vi "draw.notes.vi"(8 "error in (no error)":errorcluster, 11 "midi-ui in":refnum<class "midi-ui.lvclass">) -> (0 "error out":errorcluster, 3 "midi-ui out":refnum<class "midi-ui.lvclass">)   [LabVIEW 2020, in "midi-ui.lvclass"]
uses:
  midi-ui.lvclass
  midi-ui.lvclass/midi-ui.ctl
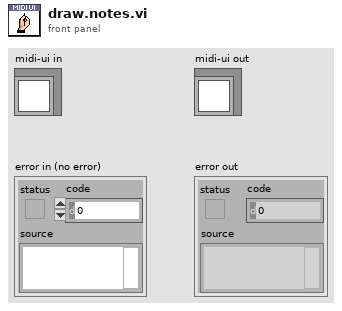
[diagram p1: front panel]
types:
  T1 = map{string, cluster{"Note On":picture, "Note Off":picture}}
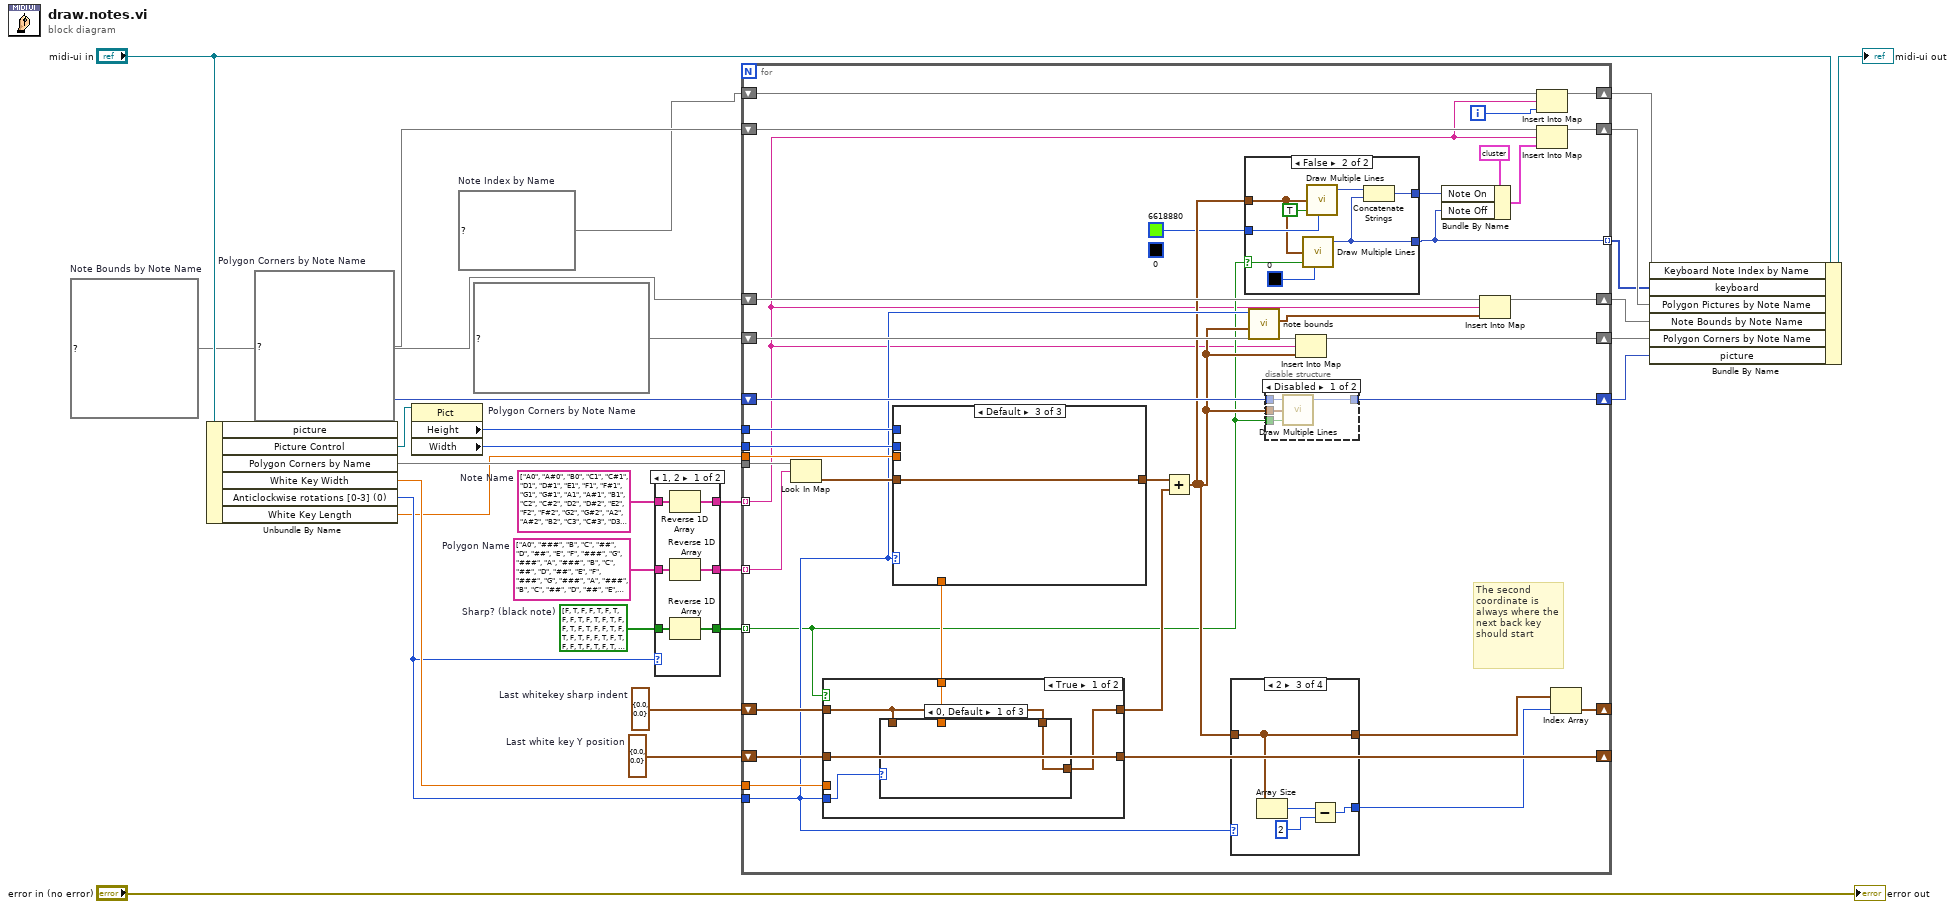
[diagram p0: block diagram]
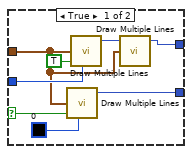
[diagram p4: hidden frame]
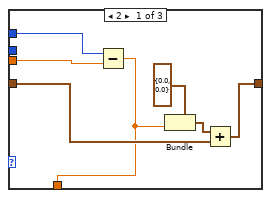
[diagram p5: hidden frame]
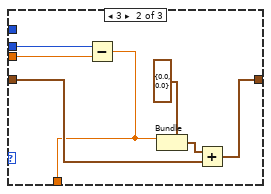
[diagram p6: hidden frame]
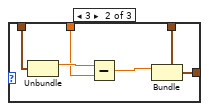
[diagram p7: hidden frame]
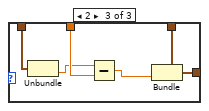
[diagram p8: hidden frame]
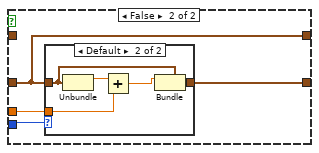
[diagram p9: hidden frame]
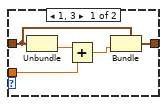
[diagram p10: hidden frame]
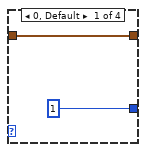
[diagram p11: hidden frame]
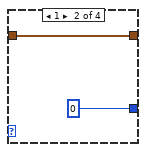
[diagram p12: hidden frame]
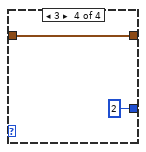
[diagram p13: hidden frame]
diagram:
  w2 = map{string, i32} {}  # Note Index by Name
  w5 = T1 {}  # Polygon Corners by Note Name
  w7 = map{string, cluster{"max":dbl, "min":dbl}} {}  # Note Bounds by Note Name
  w22 = bool[] [FALSE, TRUE, FALSE, FALSE, TRUE, FALSE, TRUE, FALSE, FALSE, TRUE, FALSE, TRUE, FALSE, TRUE, FALSE, FALSE, TRUE, FALSE, TRUE, FALSE, FALSE, TRUE, FALSE, TRUE, FALSE, TRUE, FALSE, FALSE, TRUE, FALSE, TRUE, FALSE, FALSE, TRUE, FALSE, TRUE, FALSE, TRUE, FALSE, FALSE, TRUE, FALSE, TRUE, FALSE, FALSE, TRUE, FALSE, TRUE, FALSE, TRUE, FALSE, FALSE, TRUE, FALSE, TRUE, FALSE, FALSE, TRUE, FALSE, TRUE, FALSE, TRUE, FALSE, FALSE, TRUE, FALSE, TRUE, FALSE, FALSE, TRUE, FALSE, TRUE, FALSE, TRUE, FALSE, FALSE, TRUE, FALSE, TRUE, FALSE, FALSE, TRUE, FALSE, TRUE, FALSE, TRUE, FALSE, FALSE]  # Sharp? (black note)
  w23 = string[] ["A0", "###", "B", "C", "##", "D", "##", "E", "F", "###", "G", "###", "A", "###", "B", "C", "##", "D", "##", "E", "F", "###", "G", "###", "A", "###", "B", "C", "##", "D", "##", "E", "F", "###", "G", "###", "A", "###", "B", "C", "##", "D", "##", "E", "F", "###", "G", "###", "A", "###", "B", "C", "##", "D", "##", "E", "F", "###", "G", "###", "A", "###", "B", "C", "##", "D", "##", "E", "F", "###", "G", "###", "A", "###", "B", "C", "##", "D", "##", "E", "F", "###", "G", "###", "A", "###", "B", "C8"]  # Polygon Name
  w24 = string[] ["A0", "A#0", "B0", "C1", "C#1", "D1", "D#1", "E1", "F1", "F#1", "G1", "G#1", "A1", "A#1", "B1", "C2", "C#2", "D2", "D#2", "E2", "F2", "F#2", "G2", "G#2", "A2", "A#2", "B2", "C3", "C#3", "D3", "D#3", "E3", "F3", "F#3", "G3", "G#3", "A3", "A#3", "B3", "C4", "C#4", "D4", "D#4", "E4", "F4", "F#4", "G4", "G#4", "A4", "A#4", "B4", "C5", "C#5", "D5", "D#5", "E5", "F5", "F#5", "G5", "G#5", "A5", "A#5", "B5", "C6", "C#6", "D6", "D#6", "E6", "F6", "F#6", "G6", "G#6", "A6", "A#6", "B6", "C7", "C#7", "D7", "D#7", "E7", "F7", "F#7", "G7", "G#7", "A7", "A#7", "B7", "C8"]  # Note Name
  w27 = map{string, cluster{"x":dbl, "y":dbl}[]} {}  # Polygon Corners by Note Name
  w28 = cluster{"x":dbl, "y":dbl} {"x"=0.0, "y"=0.0}  # Last whitekey sharp indent
  w29 = cluster{"x":dbl, "y":dbl} {"x"=0.0, "y"=0.0}  # Last white key Y position
  n1 = Unbundle By Name("midi-ui in") -> ("picture"=w9:picture, "Picture Control"=w13:refnum<vi>, "Polygon Corners by Name"=w26:map{string, cluster{"x":dbl, "y":dbl}[]}, "White Key Width"=w20:dbl, "Anticlockwise rotations [0-3] (0)"=w16:i32, "White Key Length"=w11:dbl)
  n2 = property class="Pict"(reference=w13) -> ("Height"=w12:u32, "Width"=w10:u32)  [unwired: 1 in, 2 out]
  n3 = case shown="1, 2" w16 {
    tunnel: w24 -> [w35 w38]
    tunnel: w23 -> [w34 w37]
    tunnel: w22 -> [w33 w36]
    tunnel: [w32 w38] -> w19
    tunnel: [w31 w37] -> w18
    tunnel: [w30 w36] -> w17
    frame 1, 2 {
      n4 = Reverse 1D Array(array=w35) -> (reversed array=w32:string[])
      n5 = Reverse 1D Array(array=w34) -> (reversed array=w31:string[])
      n6 = Reverse 1D Array(array=w33) -> (reversed array=w30:bool[])
    }
    frame Default {
    }
  }
  n7 = for {
    tunnel: w26 -> [w74]
    shift-right: [w64] -> w8
    shift-left: w9 -> [w75]
    tunnel: w19 -> [w42] mode=indexing
    shift-right: [w73] -> _
    shift-left: w29 -> [w72]
    shift-right: [w69] -> _
    shift-left: w28 -> [w70]
    shift-right: [w67] -> w15
    shift-left: w27 -> [w68]
    tunnel: w18 -> [w66] mode=indexing
    tunnel: w17 -> [w45] mode=indexing
    tunnel: w20 -> [w65]
    tunnel: w16 -> [w52]
    tunnel: w12 -> [w61]
    tunnel: w11 -> [w60]
    tunnel: w10 -> [w59]
    shift-right: [w54] -> w6
    shift-left: w7 -> [w55]
    shift-right: [w51] -> w4
    shift-left: w5 -> [w50]
    tunnel: [w39] -> w3 mode=indexing
    shift-right: [w43] -> w1
    shift-left: w2 -> [w44]
    i -> [w41]
    (unwired) u32 0 ("color(black)")
    # "The second coordinate is always where the next back key should start"
    n8 = Look In Map(map=w74, key=w66) -> (value=w57:cluster{"x":dbl, "y":dbl}[])  [unwired: 1 in, 1 out]
    n9 = case shown="Default" w52 {
      tunnel: [w98 w106 w111] -> w62
      tunnel: w57 -> [w100 w108 w111]
      tunnel: w61 -> [w103 _ _]
      tunnel: w60 -> [w102 w110 _]
      tunnel: w59 -> [_ w105 _]
      tunnel: [w97 w104 _] -> w56
      frame 2 {
        n10 = Subtract(x=w103, y=w102) -> (x-y=w97:dbl)
        n11 = Bundle(cluster=cluster{"x":dbl, "y":dbl} {"x"=0.0, "y"=0.0} ("coordinate"), "y"=w97) -> (w101:cluster{"x":dbl, "y":dbl})  [unwired: 1 in]
        n12 = Add(x=w101, y=w100) -> (x+y=w98:cluster{"x":dbl, "y":dbl}[])
      }
      frame 3 {
        n13 = Subtract(x=w105, y=w110) -> (x-y=w104:dbl)
        n14 = Bundle(cluster=cluster{"x":dbl, "y":dbl} {"x"=0.0, "y"=0.0} ("coordinate"), "x"=w104) -> (w109:cluster{"x":dbl, "y":dbl})  [unwired: 1 in]
        n15 = Add(x=w109, y=w108) -> (x+y=w106:cluster{"x":dbl, "y":dbl}[])
      }
      frame Default {
      }
    }
    n16 = case shown="True" w45 {
      tunnel: w72 -> [w116 w132]
      tunnel: [w116 w133] -> w73
      tunnel: [w114 w132] -> w71
      tunnel: w70 -> [w113 _]
      tunnel: w65 -> [_ w131]
      tunnel: w52 -> [w115 w130]
      tunnel: w56 -> [w112 _]
      frame True {
        n17 = case shown="0, Default" w115 {
          tunnel: w113 -> [w117 w123 w129]
          tunnel: [w117 w122 w128] -> w114
          tunnel: w113 -> [_ w121 w127]
          tunnel: w112 -> [_ w118 w126]
          frame 0, Default {
          }
          frame 3 {
            n18 = Unbundle(w121) -> ("x"=w120:dbl)  [unwired: 1 out]
            n19 = Subtract(x=w120, y=w118) -> (x-y=w119:dbl)
            n20 = Bundle(cluster=w123, "x"=w119) -> (w122:cluster{"x":dbl, "y":dbl})  [unwired: 1 in]
          }
          frame 2 {
            n21 = Unbundle(w127) -> ("y"=w125:dbl)  [unwired: 1 out]
            n22 = Subtract(x=w125, y=w126) -> (x-y=w124:dbl)
            n23 = Bundle(cluster=w129, "y"=w124) -> (w128:cluster{"x":dbl, "y":dbl})  [unwired: 1 in]
          }
        }
      }
      frame False {
        n24 = case shown="Default" w130 {
          tunnel: [w138 w143] -> w133
          tunnel: w132 -> [w136 w139]
          tunnel: w131 -> [w137 w142]
          frame 1, 3 {
            n25 = Unbundle(w136) -> ("y"=w135:dbl)  [unwired: 1 out]
            n26 = Add(x=w135, y=w137) -> (x+y=w134:dbl)
            n27 = Bundle(cluster=w136, "y"=w134) -> (w138:cluster{"x":dbl, "y":dbl})  [unwired: 1 in]
          }
          frame Default {
            n28 = Unbundle(w139) -> ("x"=w141:dbl)  [unwired: 1 out]
            n29 = Add(x=w141, y=w142) -> (x+y=w140:dbl)
            n30 = Bundle(cluster=w139, "x"=w140) -> (w143:cluster{"x":dbl, "y":dbl})  [unwired: 1 in]
          }
        }
      }
    }
    n31 = Add(x=w62, y=w71) -> (x+y=w48:cluster{"x":dbl, "y":dbl}[])
    n32 = case shown="2" w52 {
      tunnel: [1 0 w148 2] -> w63
      tunnel: [w144 w146 w151 w152] -> w58
      tunnel: w48 -> [w144 w146 w151 w152]
      frame 0, Default {
      }
      frame 1 {
      }
      frame 2 {
        n33 = Array Size(array=w151) -> (size(s)=w150:i32)
        n34 = Subtract(x=w150, y=2) -> (x-y=w148:i32)
      }
      frame 3 {
      }
    }
    n35 = case shown="False" w45 {
      selector: w45 -> [w85 w94]
      tunnel: w48 -> [w81 w92]
      tunnel: u32 6618880 ("color(black)") -> [w88 w96]
      tunnel: [w82 w89] -> w40
      tunnel: [w87 w90] -> w39
      frame True {
        n36 = call <vilib>:"Draw Multiple Lines.vi"("line endpoints"=w81, "fill?(F)"=w85, "color(black)"=u32 0) -> ("new picture"=w87:picture)  [unwired: 6 in]
        n37 = call <vilib>:"Draw Multiple Lines.vi"("line endpoints"=w81, "fill?(F)"=TRUE, "color(black)"=w88) -> ("new picture"=w83:picture)  [unwired: 6 in]
        n38 = call <vilib>:"Draw Multiple Lines.vi"("picture"=w83, "line endpoints"=w81) -> ("new picture"=w82:picture)  [unwired: 7 in]
      }
      frame False {
        n39 = call <vilib>:"Draw Multiple Lines.vi"("line endpoints"=w92, "fill?(F)"=w94, "color(black)"=u32 0) -> ("new picture"=w90:picture)  [unwired: 6 in]
        n40 = call <vilib>:"Draw Multiple Lines.vi"("line endpoints"=w92, "fill?(F)"=TRUE, "color(black)"=w96) -> ("new picture"=w91:picture)  [unwired: 6 in]
        n41 = Concatenate Strings(w91, w90) -> (w89:picture)
      }
    }
    n42 = call "note bounds.vi"("Note Polygone"=w48, "Anticlockwise rotations [0-3] (0)"=w52) -> ("Bounds"=w53:cluster{"Max":i16, "Min":i16})  [unwired: 9 in]
    n43 = disable-structure shown="Disabled" {
      disable-tunnel: w75 -> [w79 w80]
      disable-tunnel: [w78 w80] -> w64
      disable-tunnel: w48 -> [w77 _]
      disable-tunnel: w45 -> [w76 _]
      frame Disabled {
        n44 = call <vilib>:"Draw Multiple Lines.vi"("picture"=w79, "line endpoints"=w77, "fill?(F)"=w76) -> ("new picture"=w78:picture)  [unwired: 6 in]
      }
      frame Enabled {
      }
    }
    n45 = Insert Into Map(map in=w68, key=w42, value=w48) -> (map out=w67:map{string, cluster{"x":dbl, "y":dbl}[]})  [unwired: 2 out]
    n46 = Bundle By Name(cluster=cluster{"Note On":picture, "Note Off":picture} {"Note On"=bytes[0], "Note Off"=bytes[0]} ("value"), "Note On"=w40, "Note Off"=w39) -> (w46:cluster{"Note On":picture, "Note Off":picture})
    n47 = Insert Into Map(map in=w55, key=w42, value=w53) -> (map out=w54:map{string, cluster{"max":dbl, "min":dbl}})  [unwired: 2 out]
    n48 = Insert Into Map(map in=w44, key=w42, value=w41) -> (map out=w43:map{string, i32})  [unwired: 2 out]
    n49 = Insert Into Map(map in=w50, key=w42, value=w46) -> (map out=w51:T1)  [unwired: 2 out]
    n50 = Index Array(array=w58, index=w63) -> (element=w69:cluster{"x":dbl, "y":dbl})
  }
  n51 = Bundle By Name(cluster="midi-ui in", "Keyboard Note Index by Name"=w1, "keyboard"=w3, "Polygon Pictures by Note Name"=w4, "Note Bounds by Note Name"=w6, "Polygon Corners by Note Name"=w15, "picture"=w8) -> (→"midi-ui out":refnum<class "midi-ui.lvclass">)
  "error out" <- "error in (no error)"
